vi "Lab Panel V4.84.vi"() -> ()   [LabVIEW 2013] (continued)
                      frame False {
                      }
                      frame True {
                        n2685 = stacked-sequence {
                          tunnel: w4622 -> [w4630 _]
                          tunnel: w4621 -> [w4629 _]
                          tunnel: w4620 -> [w4628 _]
                          tunnel: w4619 -> [w4627 _]
                          tunnel: w4618 -> [w4626 _]
                          tunnel: w4617 -> [w4625 _]
                          frame #0 {
                            n2686 = call "sub vi - send mail with attach v5.vi"("TO:"=w4630, "subject"=w4628, "from"=w4626, "out going server"=w4627, "message"=w4629) -> ("error out"=w4624:errorcluster)  [unwired: 10 in]
                            n2687 = Bundle(cluster=w4625, "mail error"=w4624) -> (w4623:T6)  [unwired: 6 in]
                            n2688 = local write "MAIL SETTINGS"(w4623) -> ()
                          }
                          frame #1 {
                            n2689 = local write "mail control"("") -> ()
                            n2690 = local write "Send Mail Now"(FALSE) -> ()
                          }
                        }
                      }
                    }
                  }
                }
              }
            }
          }
          frame #18 {
            # "save jig cycle values once all run switches are off"
            n2691 = stacked-sequence {
              tunnel: w4642 -> [_ w4671]
              tunnel: w4641 -> [_ w4670]
              tunnel: w4640 -> [_ w4669]
              tunnel: w4639 -> [_ w4668]
              tunnel: w4638 -> [_ w4667]
              tunnel: w4637 -> [_ w4666]
              tunnel: w4636 -> [_ w4665]
              tunnel: w4635 -> [_ w4664]
              tunnel: w4634 -> [_ w4663]
              tunnel: w4633 -> [_ w4662]
              frame #0 {
              }
              frame #1 {
                n2692 = Not(x=w4662) -> (.not. x?=w4645:bool)
                n2693 = Not(x=w4670) -> (.not. x?=w4660:bool)
                n2694 = Not(x=w4667) -> (.not. x?=w4655:bool)
                n2695 = Not(x=w4665) -> (.not. x?=w4651:bool)
                n2696 = Not(x=w4663) -> (.not. x?=w4647:bool)
                n2697 = Not(x=w4671) -> (.not. x?=w4661:bool)
                n2698 = Not(x=w4669) -> (.not. x?=w4659:bool)
                n2699 = Not(x=w4666) -> (.not. x?=w4653:bool)
                n2700 = Not(x=w4668) -> (.not. x?=w4657:bool)
                n2701 = Not(x=w4664) -> (.not. x?=w4649:bool)
                n2702 = local read "Save JC"() -> (w4673:bool)
                n2703 = And(x=w4661, y=w4660) -> (x .and. y?=w4658:bool)
                n2704 = And(x=w4658, y=w4659) -> (x .and. y?=w4656:bool)
                n2705 = And(x=w4656, y=w4657) -> (x .and. y?=w4654:bool)
                n2706 = And(x=w4654, y=w4655) -> (x .and. y?=w4652:bool)
                n2707 = And(x=w4652, y=w4653) -> (x .and. y?=w4650:bool)
                n2708 = And(x=w4650, y=w4651) -> (x .and. y?=w4648:bool)
                n2709 = And(x=w4648, y=w4649) -> (x .and. y?=w4646:bool)
                n2710 = And(x=w4646, y=w4647) -> (x .and. y?=w4644:bool)
                n2711 = And(x=w4644, y=w4645) -> (x .and. y?=w4643:bool)
                n2712 = And(x=w4643, y=w4673) -> (x .and. y?=w4672:bool)
                n2713 = case shown="True" w4672 {
                  tunnel: w4643 -> [w4674 _]
                  frame False {
                    n2714 = case shown="False" w4674 {
                      frame False {
                        n2715 = local write "Save JC"(TRUE) -> ()
                      }
                      frame True {
                      }
                    }
                  }
                  frame True {
                    n2716 = stacked-sequence {
                      frame #0 {
                        n2717 = String To Path(string="c:\\crabtree\\Jig Cycles\\") -> (path=w4686:path)
                        n2718 = Build Path(base path=w4686, name or relative path="jigcycles.bin") -> (appended path=w4684:path)
                        n2719 = Create Folder(path (use dialog)=w4686) -> (error out=w4688:errorcluster)  [unwired: 2 in, 2 out]
                        n2720 = local read "JIG RELAY CYCLES"() -> (w4678:T7)
                        n2721 = call <vilib>:"Clear Errors.vi"("error in (no error)"=w4688) -> ()  [unwired: 6 in, 1 out]
                        n2722 = local write "Save JC"(FALSE) -> ()
                        n2723 = Open/Create/Replace File(file path (use dialog)=w4684, operation (0:open)=T19."replace or create") -> (refnum out=w4682:refnum<file>, error out=w4683:errorcluster)  [unwired: 4 in, 1 out]
                        n2724 = Write to Binary File(file (use dialog)=w4682, data=w4678, error in=w4683) -> (refnum out=w4681:refnum<file>, error out=w4680:errorcluster)  [unwired: 3 in, 1 out]
                        n2725 = Close File(refnum=w4681, error in=w4680) -> (error out=w4679:errorcluster)  [unwired: 1 out]
                        n2726 = local write "data file error"(w4679) -> ()
                      }
                      frame #1 {
                        n2727 = local read "JIG RELAY CYCLES"() -> (w4711:T7)
                        n2728 = Unbundle By Name(w4711) -> ("LAB01-1"=w4706:dbl, "LAB01-2"=w4705:dbl, "LAB02-1"=w4703:dbl, "LAB02-2"=w4702:dbl, "LAB03-1"=w4700:dbl, "LAB03-2"=w4697:dbl, "LAB04-1"=w4696:dbl, "LAB04-2"=w4694:dbl, "LAB05-1"=w4692:dbl, "LAB05-2"=w4690:dbl)
                        n2729 = stacked-sequence {
                          tunnel: w4706 -> [w4714 _ _ _ _ _ _ _ _ _]
                          tunnel: 1000000 -> [w4717 w4727 w4737 w4747 w4757 w4767 w4777 w4787 w4797 w4807]
                          tunnel: [w4715 _ _ _ _ _ _ _ _ _] -> w4709
                          tunnel: "TEST STATION HAS REACHED 1 MILLION CYCLES, REPLACE  CONTROL RELAYS" -> [w4713 w4725 w4735 w4745 w4755 w4765 w4775 w4785 w4795 w4805]
                          tunnel: [_ w4724 _ _ _ _ _ _ _ _] -> w4707
                          tunnel: w4705 -> [_ w4723 _ _ _ _ _ _ _ _]
                          tunnel: [_ _ w4734 _ _ _ _ _ _ _] -> w4704
                          tunnel: w4703 -> [_ _ w4733 _ _ _ _ _ _ _]
                          tunnel: w4702 -> [_ _ _ w4744 _ _ _ _ _ _]
                          tunnel: [_ _ _ w4743 _ _ _ _ _ _] -> w4701
                          tunnel: w4700 -> [_ _ _ _ w4754 _ _ _ _ _]
                          tunnel: [_ _ _ _ w4753 _ _ _ _ _] -> w4699
                          tunnel: [_ _ _ _ _ w4764 _ _ _ _] -> w4698
                          tunnel: w4697 -> [_ _ _ _ _ w4763 _ _ _ _]
                          tunnel: w4696 -> [_ _ _ _ _ _ w4774 _ _ _]
                          tunnel: [_ _ _ _ _ _ w4773 _ _ _] -> w4695
                          tunnel: w4694 -> [_ _ _ _ _ _ _ w4784 _ _]
                          tunnel: [_ _ _ _ _ _ _ w4783 _ _] -> w4693
                          tunnel: w4692 -> [_ _ _ _ _ _ _ _ w4794 _]
                          tunnel: [_ _ _ _ _ _ _ _ w4793 _] -> w4691
                          tunnel: w4690 -> [_ _ _ _ _ _ _ _ _ w4804]
                          tunnel: [_ _ _ _ _ _ _ _ _ w4803] -> w4689
                          frame #0 {
                            n2730 = Greater?(x=w4714, y=w4717) -> (0:w4716:bool)
                            n2731 = case shown="True" w4716 {
                              tunnel: [w4718 0] -> w4715
                              tunnel: w4714 -> [w4718 _]
                              tunnel: w4713 -> [_ w4719]
                              frame False {
                              }
                              frame True {
                                n2732 = Concatenate Strings("LA01-1 ", w4719) -> (w4722:string)
                                n2733 = One Button Dialog(message=w4722) -> ()  [unwired: 1 in, 1 out]
                              }
                            }
                          }
                          frame #1 {
                            n2734 = Greater?(x=w4723, y=w4727) -> (0:w4726:bool)
                            n2735 = case shown="True" w4726 {
                              tunnel: [w4728 0] -> w4724
                              tunnel: w4723 -> [w4728 _]
                              tunnel: w4725 -> [_ w4729]
                              frame False {
                              }
                              frame True {
                                n2736 = Concatenate Strings("LA01-2 ", w4729) -> (w4732:string)
                                n2737 = One Button Dialog(message=w4732) -> ()  [unwired: 1 in, 1 out]
                              }
                            }
                          }
                          frame #2 {
                            n2738 = Greater?(x=w4733, y=w4737) -> (0:w4736:bool)
                            n2739 = case shown="True" w4736 {
                              tunnel: [w4738 0] -> w4734
                              tunnel: w4733 -> [w4738 _]
                              tunnel: w4735 -> [_ w4739]
                              frame False {
                              }
                              frame True {
                                n2740 = Concatenate Strings("LA02-1 ", w4739) -> (w4742:string)
                                n2741 = One Button Dialog(message=w4742) -> ()  [unwired: 1 in, 1 out]
                              }
                            }
                          }
                          frame #3 {
                            n2742 = Greater?(x=w4744, y=w4747) -> (0:w4746:bool)
                            n2743 = case shown="True" w4746 {
                              tunnel: [w4748 0] -> w4743
                              tunnel: w4744 -> [w4748 _]
                              tunnel: w4745 -> [_ w4749]
                              frame False {
                              }
                              frame True {
                                n2744 = Concatenate Strings("LA02-2 ", w4749) -> (w4752:string)
                                n2745 = One Button Dialog(message=w4752) -> ()  [unwired: 1 in, 1 out]
                              }
                            }
                          }
                          frame #4 {
                            n2746 = Greater?(x=w4754, y=w4757) -> (0:w4756:bool)
                            n2747 = case shown="True" w4756 {
                              tunnel: [w4758 0] -> w4753
                              tunnel: w4754 -> [w4758 _]
                              tunnel: w4755 -> [_ w4759]
                              frame False {
                              }
                              frame True {
                                n2748 = Concatenate Strings("LA03-1 ", w4759) -> (w4762:string)
                                n2749 = One Button Dialog(message=w4762) -> ()  [unwired: 1 in, 1 out]
                              }
                            }
                          }
                          frame #5 {
                            n2750 = Greater?(x=w4763, y=w4767) -> (0:w4766:bool)
                            n2751 = case shown="True" w4766 {
                              tunnel: [w4768 0] -> w4764
                              tunnel: w4763 -> [w4768 _]
                              tunnel: w4765 -> [_ w4769]
                              frame False {
                              }
                              frame True {
                                n2752 = Concatenate Strings("LA03-2 ", w4769) -> (w4772:string)
                                n2753 = One Button Dialog(message=w4772) -> ()  [unwired: 1 in, 1 out]
                              }
                            }
                          }
                          frame #6 {
                            n2754 = Greater?(x=w4774, y=w4777) -> (0:w4776:bool)
                            n2755 = case shown="True" w4776 {
                              tunnel: [w4778 0] -> w4773
                              tunnel: w4774 -> [w4778 _]
                              tunnel: w4775 -> [_ w4779]
                              frame False {
                              }
                              frame True {
                                n2756 = Concatenate Strings("LA04-1 ", w4779) -> (w4782:string)
                                n2757 = One Button Dialog(message=w4782) -> ()  [unwired: 1 in, 1 out]
                              }
                            }
                          }
                          frame #7 {
                            n2758 = Greater?(x=w4784, y=w4787) -> (0:w4786:bool)
                            n2759 = case shown="True" w4786 {
                              tunnel: [w4788 0] -> w4783
                              tunnel: w4784 -> [w4788 _]
                              tunnel: w4785 -> [_ w4789]
                              frame False {
                              }
                              frame True {
                                n2760 = Concatenate Strings("LA04-2 ", w4789) -> (w4792:string)
                                n2761 = One Button Dialog(message=w4792) -> ()  [unwired: 1 in, 1 out]
                              }
                            }
                          }
                          frame #8 {
                            n2762 = Greater?(x=w4794, y=w4797) -> (0:w4796:bool)
                            n2763 = case shown="True" w4796 {
                              tunnel: [w4798 0] -> w4793
                              tunnel: w4794 -> [w4798 _]
                              tunnel: w4795 -> [_ w4799]
                              frame False {
                              }
                              frame True {
                                n2764 = Concatenate Strings("LA05-1 ", w4799) -> (w4802:string)
                                n2765 = One Button Dialog(message=w4802) -> ()  [unwired: 1 in, 1 out]
                              }
                            }
                          }
                          frame #9 {
                            n2766 = Greater?(x=w4804, y=w4807) -> (0:w4806:bool)
                            n2767 = case shown="True" w4806 {
                              tunnel: [w4808 0] -> w4803
                              tunnel: w4804 -> [w4808 _]
                              tunnel: w4805 -> [_ w4809]
                              frame False {
                              }
                              frame True {
                                n2768 = Concatenate Strings("LA05-2 ", w4809) -> (w4812:string)
                                n2769 = One Button Dialog(message=w4812) -> ()  [unwired: 1 in, 1 out]
                              }
                            }
                          }
                        }
                        n2770 = Bundle By Name(cluster=w4711, "LAB01-1"=w4709, "LAB01-2"=w4707, "LAB02-1"=w4704, "LAB02-2"=w4701, "LAB03-1"=w4699, "LAB03-2"=w4698, "LAB04-1"=w4695, "LAB04-2"=w4693, "LAB05-1"=w4691, "LAB05-2"=w4689) -> (w4710:T7)
                        n2771 = local write "JIG RELAY CYCLES"(w4710) -> ()
                      }
                    }
                  }
                }
              }
            }
          }
          frame #19 {
            # "get temperature values"
            n2772 = local read "simulate"() -> (w4826:bool)
            n2773 = local read "Panel #"() -> (w4813:dbl)
            n2774 = local read "Temp Test Cal"() -> (w4823:dbl)
            n2775 = stacked-sequence {
              seq-local: [w4827 _ _ _ _ _] -> [_ w4870 w4926 w4980 w5035 w5090]
              tunnel: w4826 -> [_ w4879 w4934 w4989 w5044 w5099]
              tunnel: T12 {"1  (A) cal"=1.0, "1 (V) cal"=1.0, "1 (PF) cal"=1.0, "1 (TL) cal"=1.0, "1 (TN) cal"=1.0, "2 (A) cal"=1.0, "2 (V) cal"=1.0, "2 (PF) cal"=1.0, "2 (TL) cal"=1.0, "2 (TN) cal"=1.0} ("CAL LAB01") -> [_ w4878 w4933 w4988 w5043 w5098]
              tunnel: w4824 -> [_ w4877 _ _ _ _]
              tunnel: w4823 -> [_ w4876 w4932 w4987 w5042 w5097]
              tunnel: w4822 -> [_ w4875 _ _ _ _]
              tunnel: w4821 -> [_ _ w4931 _ _ _]
              tunnel: w4820 -> [_ _ w4930 _ _ _]
              tunnel: w4819 -> [_ _ _ w4986 _ _]
              tunnel: w4818 -> [_ _ _ w4985 _ _]
              tunnel: w4817 -> [_ _ _ _ w5041 _]
              tunnel: w4816 -> [_ _ _ _ w5040 _]
              tunnel: w4815 -> [_ _ _ _ _ w5096]
              tunnel: w4814 -> [_ _ _ _ _ w5095]
              tunnel: w4813 -> [_ w4874 w4928 w4984 w5039 w5094]
              frame #0 {
                n2776 = local read "Select COM port"() -> (w4831:refnum<visa-resource-name>)
                "COM port" <- w4831
                n2777 = local read "jig cycle"() -> (w4832:dbl)
                n2778 = local read "on loops"() -> (w4834:dbl)
                n2779 = global write "Global 1.vi" "tmp dly lps"("Temp Delay Lps") -> ()
                n2780 = global write "Global 1.vi" "dly value"("Temp Value") -> ()
                n2781 = Add(x=w4834, y=3) -> (x+y=w4835:dbl)
                n2782 = global write "Global 1.vi" "COM port"(w4831) -> ()
                n2783 = Equal?(x=w4832, y=w4835) -> (x = y?=w4827:bool)
                n2784 = local read "Panel #"() -> (w4828:dbl)
                n2785 = case shown="True" w4827 {
                  tunnel: w4828 -> [_ w4837]
                  frame False {
                  }
                  frame True {
                    n2786 = stacked-sequence {
                      tunnel: w4837 -> [w4840 w4868]
                      frame #0 {
                        n2787 = local read "simulate"() -> (w4838:bool)
                        n2788 = case shown="3" w4840 {
                          tunnel: 1.0 -> [_ w4845 w4847 w4853 w4857 w4862]
                          tunnel: w4838 -> [_ w4841 w4846 w4851 w4858 w4861]
                          frame 0, Default {
                          }
                          frame 1 {
                            w4843 = FALSE
                            n2789 = call "sub vi - GET ALL TEMP v5.vi"("LA01-EN"=TRUE, "simulate"=w4841, "LA02-EN"=w4843, "LA03-EN"=w4843, "LA04-EN"=w4843, "LA05-EN"=w4843, "Gen Cal Value"=w4845) -> ("LA01 TEMP"=w4842:T22)  [unwired: 3 in, 5 out]
                            n2790 = local write "LAB01 TEMP"(w4842) -> ()
                          }
                          frame 2 {
                            w4848 = FALSE
                            n2791 = call "sub vi - GET ALL TEMP v5.vi"("LA01-EN"=w4848, "simulate"=w4846, "LA02-EN"=TRUE, "LA03-EN"=w4848, "LA04-EN"=w4848, "LA05-EN"=w4848, "Gen Cal Value"=w4847) -> ("LA02 TEMP"=w4850:T22)  [unwired: 3 in, 5 out]
                            n2792 = local write "LAB02 TEMP"(w4850) -> ()
                          }
                          frame 3 {
                            w4854 = FALSE
                            n2793 = call "sub vi - GET ALL TEMP v5.vi"("LA01-EN"=w4854, "simulate"=w4851, "LA02-EN"=w4854, "LA03-EN"=TRUE, "LA04-EN"=w4854, "LA05-EN"=w4854, "Gen Cal Value"=w4853) -> ("LA03 TEMP"=w4852:T22)  [unwired: 3 in, 5 out]
                            n2794 = local write "LAB03 TEMP"(w4852) -> ()
                          }
                          frame 4 {
                            w4859 = FALSE
                            n2795 = call "sub vi - GET ALL TEMP v5.vi"("LA01-EN"=w4859, "simulate"=w4858, "LA02-EN"=w4859, "LA03-EN"=w4859, "LA04-EN"=TRUE, "LA05-EN"=w4859, "Gen Cal Value"=w4857) -> ("LA04 TEMP"=w4856:T22)  [unwired: 3 in, 5 out]
                            n2796 = local write "LAB04 TEMP"(w4856) -> ()
                          }
                          frame 5 {
                            w4864 = FALSE
                            n2797 = call "sub vi - GET ALL TEMP v5.vi"("LA01-EN"=w4864, "simulate"=w4861, "LA02-EN"=w4864, "LA03-EN"=w4864, "LA04-EN"=w4864, "LA05-EN"=TRUE, "Gen Cal Value"=w4862) -> ("LA05 TEMP"=w4863:T22)  [unwired: 3 in, 5 out]
                            n2798 = local write "LAB05 TEMP"(w4863) -> ()
                          }
                        }
                      }
                      frame #1 {
                        n2799 = Greater Or Equal?(x=w4868, y=5) -> (x >= y?=w4866:bool)
                        n2800 = case shown="True" w4866 {
                          frame False {
                          }
                          frame True {
                            n2801 = local write "Panel #"(0) -> ()
                          }
                        }
                      }
                    }
                    n2802 = local write "TEMP"(TRUE) -> ()
                  }
                }
              }
              frame #1 {
                n2803 = Equal?(x=w4874, y=1) -> (x = y?=w4872:bool)
                n2804 = And(x=w4872, y=w4870) -> (x .and. y?=w4871:bool)
                n2805 = case shown="True" w4871 {
                  tunnel: w4879 -> [_ w4892]
                  tunnel: w4878 -> [_ w4891]
                  tunnel: w4877 -> [_ w4889]
                  tunnel: w4876 -> [_ w4885]
                  tunnel: w4875 -> [_ w4880]
                  frame False {
                  }
                  frame True {
                    n2806 = case shown="False" w4892 {
                      tunnel: [w4923 w4924] -> w4908
                      tunnel: w4891 -> [_ w4924]
                      frame False {
                        n2807 = local read "CAL LAB01"() -> (w4923:T12)
                      }
                      frame True {
                      }
                    }
                    n2808 = local read "LAB01 TEMP"() -> (w4898:T11)
                    n2809 = local read "TEMP LA01"() -> (w4899:T8)
                    n2810 = call "sub vi - temperature delay v2.vi"("temp values IN"=w4899, "temp signals"=w4898) -> ("T2-N"=w4894:dbl, "T2-L"=w4895:dbl, "T1-N"=w4896:dbl, "T1-L"=w4897:dbl, "temp values OUT"=w4893:T39)  [unwired: 5 in]
                    n2811 = Unbundle By Name(w4908) -> ("1 (TL) cal"=w4903:dbl, "1 (TN) cal"=w4902:dbl, "2 (TL) cal"=w4901:dbl, "2 (TN) cal"=w4900:dbl)  [unwired: 6 out]
                    n2812 = local write "TEMP LA01"(w4893) -> ()
                    n2813 = Multiply(x=w4897, y=w4903) -> (x*y=w4890:dbl)
                    n2814 = Multiply(x=w4896, y=w4902) -> (x*y=w4887:dbl)
                    n2815 = Multiply(x=w4895, y=w4901) -> (x*y=w4884:dbl)
                    n2816 = Multiply(x=w4894, y=w4900) -> (x*y=w4883:dbl)
                    n2817 = case shown="True" w4889 {
                      tunnel: w4890 -> [w4917 w4922]
                      tunnel: w4885 -> [_ w4920]
                      tunnel: [w4917 w4921] -> w4888
                      tunnel: w4887 -> [w4916 w4919]
                      tunnel: [w4916 w4918] -> w4886
                      frame False {
                      }
                      frame True {
                        n2818 = Multiply(x=w4920, y=w4919) -> (x*y=w4918:dbl)
                        n2819 = Multiply(x=w4920, y=w4922) -> (x*y=w4921:dbl)
                      }
                    }
                    n2820 = case shown="True" w4880 {
                      tunnel: w4884 -> [w4910 w4915]
                      tunnel: w4885 -> [_ w4913]
                      tunnel: [w4910 w4914] -> w4882
                      tunnel: w4883 -> [w4909 w4912]
                      tunnel: [w4909 w4911] -> w4881
                      frame False {
                      }
                      frame True {
                        n2821 = Multiply(x=w4913, y=w4912) -> (x*y=w4911:dbl)
                        n2822 = Multiply(x=w4913, y=w4915) -> (x*y=w4914:dbl)
                      }
                    }
                    n2823 = local read "SIG LAB01-2"() -> (w4905:T2)
                    n2824 = local read "SIG LAB01-1"() -> (w4907:T2)
                    n2825 = Bundle By Name(cluster=w4907, "Tmp Live"=w4888, "Tmp Neut"=w4886) -> (w4906:T2)
                    n2826 = Bundle By Name(cluster=w4905, "Tmp Live"=w4882, "Tmp Neut"=w4881) -> (w4904:T2)
                    n2827 = local write "SIG LAB01-1"(w4906) -> ()
                    n2828 = local write "SIG LAB01-2"(w4904) -> ()
                  }
                }
              }
              frame #2 {
                n2829 = Equal?(x=w4928, y=2) -> (x = y?=w4927:bool)
                n2830 = And(x=w4927, y=w4926) -> (x .and. y?=w4925:bool)
                n2831 = case shown="True" w4925 {
                  tunnel: w4934 -> [_ w4947]
                  tunnel: w4933 -> [_ w4946]
                  tunnel: w4932 -> [_ w4945]
                  tunnel: w4931 -> [_ w4936]
                  tunnel: w4930 -> [_ w4935]
                  frame False {
                  }
                  frame True {
                    n2832 = case shown="True" w4947 {
                      tunnel: [w4978 w4979] -> w4963
                      tunnel: w4946 -> [_ w4979]
                      frame False {
                        n2833 = local read "CAL LAB02"() -> (w4978:T13)
                      }
                      frame True {
                      }
                    }
                    n2834 = local read "LAB02 TEMP"() -> (w4954:T11)
                    n2835 = local read "TEMP LA02"() -> (w4953:T8)
                    n2836 = call "sub vi - temperature delay v2.vi"("temp values IN"=w4953, "temp signals"=w4954) -> ("T2-N"=w4948:dbl, "T2-L"=w4949:dbl, "T1-N"=w4950:dbl, "T1-L"=w4951:dbl, "temp values OUT"=w4952:T39)  [unwired: 5 in]
                    n2837 = Unbundle By Name(w4963) -> ("1 (TL) cal"=w4958:dbl, "1 (TN) cal"=w4957:dbl, "2 (TL) cal"=w4956:dbl, "2 (TN) cal"=w4955:dbl)  [unwired: 6 out]
                    n2838 = local write "TEMP LA02"(w4952) -> ()
                    n2839 = Multiply(x=w4951, y=w4958) -> (x*y=w4944:dbl)
                    n2840 = Multiply(x=w4950, y=w4957) -> (x*y=w4943:dbl)
                    n2841 = Multiply(x=w4949, y=w4956) -> (x*y=w4940:dbl)
                    n2842 = Multiply(x=w4948, y=w4955) -> (x*y=w4939:dbl)
                    n2843 = case shown="True" w4936 {
                      tunnel: w4944 -> [w4972 w4977]
                      tunnel: w4945 -> [_ w4975]
                      tunnel: [w4972 w4976] -> w4942
                      tunnel: w4943 -> [w4971 w4974]
                      tunnel: [w4971 w4973] -> w4941
                      frame False {
                      }
                      frame True {
                        n2844 = Multiply(x=w4975, y=w4974) -> (x*y=w4973:dbl)
                        n2845 = Multiply(x=w4975, y=w4977) -> (x*y=w4976:dbl)
                      }
                    }
                    n2846 = case shown="True" w4935 {
                      tunnel: w4940 -> [w4965 w4970]
                      tunnel: w4945 -> [_ w4968]
                      tunnel: [w4965 w4969] -> w4938
                      tunnel: w4939 -> [w4964 w4967]
                      tunnel: [w4964 w4966] -> w4937
                      frame False {
                      }
                      frame True {
                        n2847 = Multiply(x=w4968, y=w4967) -> (x*y=w4966:dbl)
                        n2848 = Multiply(x=w4968, y=w4970) -> (x*y=w4969:dbl)
                      }
                    }
                    n2849 = local read "SIG LAB02-2"() -> (w4960:T2)
                    n2850 = local read "SIG LAB02-1"() -> (w4962:T2)
                    n2851 = Bundle By Name(cluster=w4962, "Tmp Live"=w4942, "Tmp Neut"=w4941) -> (w4961:T2)
                    n2852 = Bundle By Name(cluster=w4960, "Tmp Live"=w4938, "Tmp Neut"=w4937) -> (w4959:T2)
                    n2853 = local write "SIG LAB02-1"(w4961) -> ()
                    n2854 = local write "SIG LAB02-2"(w4959) -> ()
                  }
                }
              }
              frame #3 {
                n2855 = Equal?(x=w4984, y=3) -> (x = y?=w4981:bool)
                n2856 = And(x=w4981, y=w4980) -> (x .and. y?=w4982:bool)
                n2857 = case shown="True" w4982 {
                  tunnel: w4989 -> [_ w5002]
                  tunnel: w4988 -> [_ w5001]
                  tunnel: w4987 -> [_ w5000]
                  tunnel: w4986 -> [_ w4991]
                  tunnel: w4985 -> [_ w4990]
                  frame False {
                  }
                  frame True {
                    n2858 = case shown="False" w5002 {
                      tunnel: [w5033 w5034] -> w5018
                      tunnel: w5001 -> [_ w5034]
                      frame False {
                        n2859 = local read "CAL LAB03"() -> (w5033:T12)
                      }
                      frame True {
                      }
                    }
                    n2860 = local read "TEMP LA03"() -> (w5008:T8)
                    n2861 = local read "LAB03 TEMP"() -> (w5009:T11)
                    n2862 = call "sub vi - temperature delay v2.vi"("temp values IN"=w5008, "temp signals"=w5009) -> ("T2-N"=w5003:dbl, "T2-L"=w5004:dbl, "T1-N"=w5005:dbl, "T1-L"=w5006:dbl, "temp values OUT"=w5007:T39)  [unwired: 5 in]
                    n2863 = Unbundle By Name(w5018) -> ("1 (TL) cal"=w5013:dbl, "1 (TN) cal"=w5012:dbl, "2 (TL) cal"=w5011:dbl, "2 (TN) cal"=w5010:dbl)  [unwired: 6 out]
                    n2864 = local write "TEMP LA03"(w5007) -> ()
                    n2865 = Multiply(x=w5006, y=w5013) -> (x*y=w4999:dbl)
                    n2866 = Multiply(x=w5005, y=w5012) -> (x*y=w4998:dbl)
                    n2867 = Multiply(x=w5004, y=w5011) -> (x*y=w4995:dbl)
                    n2868 = Multiply(x=w5003, y=w5010) -> (x*y=w4994:dbl)
                    n2869 = case shown="True" w4990 {
                      tunnel: w4995 -> [w5020 w5025]
                      tunnel: w5000 -> [_ w5023]
                      tunnel: [w5020 w5024] -> w4993
                      tunnel: w4994 -> [w5019 w5022]
                      tunnel: [w5019 w5021] -> w4992
                      frame False {
                      }
                      frame True {
                        n2870 = Multiply(x=w5023, y=w5022) -> (x*y=w5021:dbl)
                        n2871 = Multiply(x=w5023, y=w5025) -> (x*y=w5024:dbl)
                      }
                    }
                    n2872 = case shown="True" w4991 {
                      tunnel: w4999 -> [w5027 w5032]
                      tunnel: w5000 -> [_ w5030]
                      tunnel: [w5027 w5031] -> w4997
                      tunnel: w4998 -> [w5026 w5029]
                      tunnel: [w5026 w5028] -> w4996
                      frame False {
                      }
                      frame True {
                        n2873 = Multiply(x=w5030, y=w5029) -> (x*y=w5028:dbl)
                        n2874 = Multiply(x=w5030, y=w5032) -> (x*y=w5031:dbl)
                      }
                    }
                    n2875 = local read "SIG LAB03-2"() -> (w5015:T2)
                    n2876 = local read "SIG LAB03-1"() -> (w5017:T2)
                    n2877 = Bundle By Name(cluster=w5017, "Tmp Live"=w4997, "Tmp Neut"=w4996) -> (w5016:T2)
                    n2878 = Bundle By Name(cluster=w5015, "Tmp Live"=w4993, "Tmp Neut"=w4992) -> (w5014:T2)
                    n2879 = local write "SIG LAB03-1"(w5016) -> ()
                    n2880 = local write "SIG LAB03-2"(w5014) -> ()
                  }
                }
              }
              frame #4 {
                n2881 = Equal?(x=w5039, y=4) -> (x = y?=w5036:bool)
                n2882 = And(x=w5036, y=w5035) -> (x .and. y?=w5037:bool)
                n2883 = case shown="True" w5037 {
                  tunnel: w5044 -> [_ w5057]
                  tunnel: w5043 -> [_ w5056]
                  tunnel: w5042 -> [_ w5055]
                  tunnel: w5041 -> [_ w5046]
                  tunnel: w5040 -> [_ w5045]
                  frame False {
                  }
                  frame True {
                    n2884 = case shown="False" w5057 {
                      tunnel: [w5088 w5089] -> w5073
                      tunnel: w5056 -> [_ w5089]
                      frame False {
                        n2885 = local read "CAL LAB04"() -> (w5088:T12)
                      }
                      frame True {
                      }
                    }
                    n2886 = local read "LAB04 TEMP"() -> (w5063:T11)
                    n2887 = local read "TEMP LA04"() -> (w5064:T8)
                    n2888 = call "sub vi - temperature delay v2.vi"("temp values IN"=w5064, "temp signals"=w5063) -> ("T2-N"=w5058:dbl, "T2-L"=w5059:dbl, "T1-N"=w5060:dbl, "T1-L"=w5061:dbl, "temp values OUT"=w5062:T39)  [unwired: 5 in]
                    n2889 = Unbundle By Name(w5073) -> ("1 (TL) cal"=w5068:dbl, "1 (TN) cal"=w5067:dbl, "2 (TL) cal"=w5066:dbl, "2 (TN) cal"=w5065:dbl)  [unwired: 6 out]
                    n2890 = local write "TEMP LA04"(w5062) -> ()
                    n2891 = Multiply(x=w5061, y=w5068) -> (x*y=w5054:dbl)
                    n2892 = Multiply(x=w5060, y=w5067) -> (x*y=w5053:dbl)
                    n2893 = Multiply(x=w5059, y=w5066) -> (x*y=w5050:dbl)
                    n2894 = Multiply(x=w5058, y=w5065) -> (x*y=w5049:dbl)
                    n2895 = case shown="True" w5045 {
                      tunnel: w5050 -> [w5075 w5080]
                      tunnel: w5055 -> [_ w5078]
                      tunnel: [w5075 w5079] -> w5048
                      tunnel: w5049 -> [w5074 w5077]
                      tunnel: [w5074 w5076] -> w5047
                      frame False {
                      }
                      frame True {
                        n2896 = Multiply(x=w5078, y=w5077) -> (x*y=w5076:dbl)
                        n2897 = Multiply(x=w5078, y=w5080) -> (x*y=w5079:dbl)
                      }
                    }
                    n2898 = case shown="True" w5046 {
                      tunnel: w5054 -> [w5082 w5087]
                      tunnel: w5055 -> [_ w5085]
                      tunnel: [w5082 w5086] -> w5052
                      tunnel: w5053 -> [w5081 w5084]
                      tunnel: [w5081 w5083] -> w5051
                      frame False {
                      }
                      frame True {
                        n2899 = Multiply(x=w5085, y=w5084) -> (x*y=w5083:dbl)
                        n2900 = Multiply(x=w5085, y=w5087) -> (x*y=w5086:dbl)
                      }
                    }
                    n2901 = local read "SIG LAB04-2"() -> (w5070:T2)
                    n2902 = local read "SIG LAB04-1"() -> (w5072:T2)
                    n2903 = Bundle By Name(cluster=w5072, "Tmp Live"=w5052, "Tmp Neut"=w5051) -> (w5071:T2)
                    n2904 = Bundle By Name(cluster=w5070, "Tmp Live"=w5048, "Tmp Neut"=w5047) -> (w5069:T2)
                    n2905 = local write "SIG LAB04-1"(w5071) -> ()
                    n2906 = local write "SIG LAB04-2"(w5069) -> ()
                  }
                }
              }
              frame #5 {
                n2907 = Equal?(x=w5094, y=5) -> (x = y?=w5091:bool)
                n2908 = And(x=w5091, y=w5090) -> (x .and. y?=w5092:bool)
                n2909 = case shown="True" w5092 {
                  tunnel: w5099 -> [_ w5112]
                  tunnel: w5098 -> [_ w5111]
                  tunnel: w5097 -> [_ w5110]
                  tunnel: w5096 -> [_ w5101]
                  tunnel: w5095 -> [_ w5100]
                  frame False {
                  }
                  frame True {
                    n2910 = case shown="False" w5112 {
                      tunnel: [w5143 w5144] -> w5128
                      tunnel: w5111 -> [_ w5144]
                      frame False {
                        n2911 = local read "CAL LAB05"() -> (w5143:T12)
                      }
                      frame True {
                      }
                    }
                    n2912 = local read "LAB05 TEMP"() -> (w5118:T11)
                    n2913 = local read "TEMP LA05"() -> (w5119:T8)
                    n2914 = call "sub vi - temperature delay v2.vi"("temp values IN"=w5119, "temp signals"=w5118) -> ("T2-N"=w5114:dbl, "T2-L"=w5115:dbl, "T1-N"=w5116:dbl, "T1-L"=w5117:dbl, "temp values OUT"=w5113:T39)  [unwired: 5 in]
                    n2915 = local write "TEMP LA05"(w5113) -> ()
                    n2916 = Unbundle By Name(w5128) -> ("1 (TL) cal"=w5120:dbl, "1 (TN) cal"=w5123:dbl, "2 (TL) cal"=w5122:dbl, "2 (TN) cal"=w5121:dbl)  [unwired: 6 out]
                    n2917 = Multiply(x=w5117, y=w5120) -> (x*y=w5109:dbl)
                    n2918 = Multiply(x=w5116, y=w5123) -> (x*y=w5108:dbl)
                    n2919 = Multiply(x=w5115, y=w5122) -> (x*y=w5105:dbl)
                    n2920 = Multiply(x=w5114, y=w5121) -> (x*y=w5104:dbl)
                    n2921 = case shown="True" w5100 {
                      tunnel: w5105 -> [w5130 w5135]
                      tunnel: w5110 -> [_ w5133]
                      tunnel: [w5130 w5134] -> w5103
                      tunnel: w5104 -> [w5129 w5132]
                      tunnel: [w5129 w5131] -> w5102
                      frame False {
                      }
                      frame True {
                        n2922 = Multiply(x=w5133, y=w5132) -> (x*y=w5131:dbl)
                        n2923 = Multiply(x=w5133, y=w5135) -> (x*y=w5134:dbl)
                      }
                    }
                    n2924 = case shown="True" w5101 {
                      tunnel: w5109 -> [w5137 w5142]
                      tunnel: w5110 -> [_ w5140]
                      tunnel: [w5137 w5141] -> w5107
                      tunnel: w5108 -> [w5136 w5139]
                      tunnel: [w5136 w5138] -> w5106
                      frame False {
                      }
                      frame True {
                        n2925 = Multiply(x=w5140, y=w5139) -> (x*y=w5138:dbl)
                        n2926 = Multiply(x=w5140, y=w5142) -> (x*y=w5141:dbl)
                      }
                    }
                    n2927 = local read "SIG LAB05-1"() -> (w5127:T2)
                    n2928 = Bundle By Name(cluster=w5127, "Tmp Live"=w5107, "Tmp Neut"=w5106) -> (w5126:T2)
                    n2929 = local read "SIG LAB05-2"() -> (w5125:T2)
                    n2930 = Bundle By Name(cluster=w5125, "Tmp Live"=w5103, "Tmp Neut"=w5102) -> (w5124:T2)
                    n2931 = local write "SIG LAB05-1"(w5126) -> ()
                    n2932 = local write "SIG LAB05-2"(w5124) -> ()
                  }
                }
              }
            }
          }
          frame #20 {
            # "write data to display panel"
            n2933 = global write "Global display 1.vi" "TEST 5-2"(w5159) -> ()
            n2934 = global write "Global display 1.vi" "TEST 4-2"(w5161) -> ()
            n2935 = global write "Global display 1.vi" "TEST 1-2"(w5167) -> ()
            n2936 = global write "Global display 1.vi" "TEST 3-1"(w5164) -> ()
            n2937 = global write "Global display 1.vi" "TEST 5-1"(w5160) -> ()
            n2938 = global write "Global display 1.vi" "TEST 1-1"(w5168) -> ()
            n2939 = global write "Global display 1.vi" "TEST 3-2"(w5163) -> ()
            n2940 = global write "Global display 1.vi" "TEST 4-1"(w5162) -> ()
            n2941 = global write "Global display 1.vi" "TEST 2-2"(w5165) -> ()
            n2942 = global write "Global display 1.vi" "TEST 2-1"(w5166) -> ()
            n2943 = global read "Global display 3.vi" "log 1-1"() -> (→"LOG LAB01-1":string)
            n2944 = global read "Global display 3.vi" "log 3-1"() -> (→"LOG LAB03-1":string)
            n2945 = global read "Global display 3.vi" "log 1-2"() -> (→"LOG LAB01-2":string)
            n2946 = property on="Tab Control 2" class="TabCtl (strict)"() -> ("Pages"=w5158:refnum<vi>[])  [unwired: 2 in, 2 out]
            n2947 = global read "Global display 3.vi" "log 2-1"() -> (→"LOG LAB02-1":string)
            n2948 = global read "Global display 3.vi" "log 2-2"() -> (→"LOG LAB02-2":string)
            n2949 = global read "Global display 3.vi" "log 4-2"() -> (→"LOG LAB04-2":string)
            n2950 = global read "Global display 3.vi" "log 5-2"() -> (→"LOG LAB05-2":string)
            n2951 = global read "Global display 3.vi" "log 5-1"() -> (→"LOG LAB05-1":string)
            n2952 = global read "Global display 3.vi" "log 4-1"() -> (→"LOG LAB04-1":string)
            n2953 = global read "Global display 3.vi" "log 3-2"() -> (→"LOG LAB03-2":string)
            n2954 = Index Array(array=w5158, index=9) -> (element=w5156:refnum<vi>)
            n2955 = property class="Page"(reference=w5156) -> ("PageVis"=w5155:bool)  [unwired: 1 in, 2 out]
            n2956 = global write "Global display 3.vi" "admin"(w5155) -> ()
            n2957 = local read "O/I  LAB05-2"() -> (w5209:bool)
            n2958 = local read "O/I  LAB05-1"() -> (w5210:bool)
            n2959 = local read "O/I  LAB03-2"() -> (w5213:bool)
            n2960 = local read "O/I  LAB04-2"() -> (w5211:bool)
            n2961 = local read "O/I  LAB04-1"() -> (w5212:bool)
            n2962 = local read "O/I  LAB03-1"() -> (w5214:bool)
            n2963 = local read "O/I  LAB01-2"() -> (w5217:bool)
            n2964 = local read "O/I  LAB01-1"() -> (w5218:bool)
            n2965 = local read "O/I  LAB02-1"() -> (w5216:bool)
            n2966 = local read "O/I  LAB02-2"() -> (w5215:bool)
            n2967 = global write "Global display 1.vi" "5-2 O/F"(w5209) -> ()
            n2968 = global write "Global display 1.vi" "5-1 O/F"(w5210) -> ()
            n2969 = global write "Global display 1.vi" "4-1 O/F"(w5212) -> ()
            n2970 = global write "Global display 1.vi" "4-2 O/F"(w5211) -> ()
            n2971 = global write "Global display 1.vi" "3-2 O/F"(w5213) -> ()
            n2972 = global write "Global display 1.vi" "3-1 O/F"(w5214) -> ()
            n2973 = global write "Global display 1.vi" "2-2 O/F"(w5215) -> ()
            n2974 = global write "Global display 1.vi" "2-1 O/F"(w5216) -> ()
            n2975 = global write "Global display 1.vi" "1-2 O/F"(w5217) -> ()
            n2976 = global write "Global display 1.vi" "1-1 O/F"(w5218) -> ()
            n2977 = local read "run lab05-2"() -> (w5199:bool)
            n2978 = local read "run lab04-1"() -> (w5202:bool)
            n2979 = local read "run lab04-2"() -> (w5201:bool)
            n2980 = local read "run lab05-1"() -> (w5200:bool)
            n2981 = local read "run lab03-2"() -> (w5203:bool)
            n2982 = local read "run lab02-1"() -> (w5206:bool)
            n2983 = local read "run lab03-1"() -> (w5204:bool)
            n2984 = local read "run lab01-2"() -> (w5207:bool)
            n2985 = local read "run lab02-2"() -> (w5205:bool)
            n2986 = local read "run lab01-1"() -> (w5208:bool)
            n2987 = global write "Global display 1.vi" "5-2 R/S"(w5199) -> ()
            n2988 = global write "Global display 1.vi" "5-1 R/S"(w5200) -> ()
            n2989 = global write "Global display 1.vi" "4-2 R/S"(w5201) -> ()
            n2990 = global write "Global display 1.vi" "4-1 R/S"(w5202) -> ()
            n2991 = global write "Global display 1.vi" "3-2 R/S"(w5203) -> ()
            n2992 = global write "Global display 1.vi" "1-2 R/S"(w5207) -> ()
            n2993 = global write "Global display 1.vi" "2-1 R/S"(w5206) -> ()
            n2994 = global write "Global display 1.vi" "3-1 R/S"(w5204) -> ()
            n2995 = global write "Global display 1.vi" "2-2 R/S"(w5205) -> ()
            n2996 = global write "Global display 1.vi" "1-1 R/S"(w5208) -> ()
            n2997 = local read "DISP LAB04-2"() -> (w5191:T4)
            n2998 = local read "DISP LAB05-1"() -> (w5190:T4)
            n2999 = local read "DISP LAB04-1"() -> (w5192:T4)
            n3000 = local read "DISP LAB05-2"() -> (w5189:T4)
            n3001 = local read "DISP LAB03-1"() -> (w5194:T4)
            n3002 = local read "DISP LAB03-2"() -> (w5193:T4)
            n3003 = local read "DISP LAB01-2"() -> (w5197:T4)
            n3004 = local read "DISP LAB02-1"() -> (w5196:T4)
            n3005 = local read "DISP LAB02-2"() -> (w5195:T4)
            n3006 = local read "DISP LAB01-1"() -> (w5198:T4)
            n3007 = global write "Global display 2.vi" "DISP LAB05-1"(w5190) -> ()
            n3008 = global write "Global display 2.vi" "DISP LAB05-2"(w5189) -> ()
            n3009 = global write "Global display 2.vi" "DISP LAB04-2"(w5191) -> ()
            n3010 = global write "Global display 2.vi" "DISP LAB02-1"(w5196) -> ()
            n3011 = global write "Global display 2.vi" "DISP LAB02-2"(w5195) -> ()
            n3012 = global write "Global display 2.vi" "DISP LAB04-1"(w5192) -> ()
            n3013 = global write "Global display 2.vi" "DISP LAB01-2"(w5197) -> ()
            n3014 = global write "Global display 2.vi" "DISP LAB01-1"(w5198) -> ()
            n3015 = global write "Global display 2.vi" "DISP LAB03-1"(w5194) -> ()
            n3016 = global write "Global display 2.vi" "DISP LAB03-2"(w5193) -> ()
            n3017 = local read "SET LAB05-2"() -> (w5179:T5)
            n3018 = local read "SET LAB05-1"() -> (w5180:T5)
            n3019 = local read "SET LAB04-1"() -> (w5182:T5)
            n3020 = local read "SET LAB04-2"() -> (w5181:T5)
            n3021 = local read "SET LAB03-1"() -> (w5184:T5)
            n3022 = local read "SET LAB03-2"() -> (w5183:T5)
            n3023 = local read "SET LAB02-2"() -> (w5185:T5)
            n3024 = local read "SET LAB01-2"() -> (w5187:T5)
            n3025 = local read "SET LAB02-1"() -> (w5186:T5)
            n3026 = local read "SET LAB01-1"() -> (w5188:T5)
            n3027 = global write "Global display 2.vi" "SET LAB05-2"(w5179) -> ()
            n3028 = global write "Global display 2.vi" "SET LAB05-1"(w5180) -> ()
            n3029 = global write "Global display 2.vi" "SET LAB04-1"(w5182) -> ()
            n3030 = global write "Global display 2.vi" "SET LAB04-2"(w5181) -> ()
            n3031 = global write "Global display 2.vi" "SET LAB03-2"(w5183) -> ()
            n3032 = global write "Global display 2.vi" "SET LAB02-2"(w5185) -> ()
            n3033 = global write "Global display 2.vi" "SET LAB03-1"(w5184) -> ()
            n3034 = global write "Global display 2.vi" "SET LAB01-2"(w5187) -> ()
            n3035 = global write "Global display 2.vi" "SET LAB01-1"(w5188) -> ()
            n3036 = global write "Global display 2.vi" "SET LAB02-1"(w5186) -> ()
            n3037 = local read "RESULT LAB01-1"() -> (w5178:bool)
            n3038 = local read "RESULT LAB03-2"() -> (w5173:bool)
            n3039 = local read "RESULT LAB04-1"() -> (w5172:bool)
            n3040 = local read "RESULT LAB04-2"() -> (w5171:bool)
            n3041 = local read "RESULT LAB02-2"() -> (w5175:bool)
            n3042 = local read "RESULT LAB01-2"() -> (w5177:bool)
            n3043 = local read "RESULT LAB02-1"() -> (w5176:bool)
            n3044 = local read "RESULT LAB03-1"() -> (w5174:bool)
            n3045 = local read "RESULT LAB05-1"() -> (w5170:bool)
            n3046 = local read "RESULT LAB05-2"() -> (w5169:bool)
            n3047 = global write "Global display 2.vi" "RESULT LAB05-1"(w5170) -> ()
            n3048 = global write "Global display 2.vi" "RESULT LAB01-2"(w5177) -> ()
            n3049 = global write "Global display 2.vi" "RESULT LAB03-2"(w5173) -> ()
            n3050 = global write "Global display 2.vi" "RESULT LAB04-1"(w5172) -> ()
            n3051 = global write "Global display 2.vi" "RESULT LAB04-2"(w5171) -> ()
            n3052 = global write "Global display 2.vi" "RESULT LAB05-2"(w5169) -> ()
            n3053 = global write "Global display 2.vi" "RESULT LAB03-1"(w5174) -> ()
            n3054 = global write "Global display 2.vi" "RESULT LAB02-1"(w5176) -> ()
            n3055 = global write "Global display 2.vi" "RESULT LAB02-2"(w5175) -> ()
            n3056 = global write "Global display 2.vi" "RESULT LAB01-1"(w5178) -> ()
          }
          frame #21 {
            # "end main and display program"
            n3057 = Quit LabVIEW(quit? (T)="stop all") -> ()
            n3058 = global write "Global display 1.vi" "stop disp"("stop all") -> ()
          }
        }
        n3059 = node-c288() -> ()  [unwired: 1 in, 1 out]
        "loops" <- w287
      }
      n3060 = node-c288(w264) -> ()  [unwired: 1 out]
    }
  }
